vi "populate sonde row cluster from row.vi"(2 "Time Value":dbl, 7 "Initialize Initial Value Cluster":bool, 8 "error in (no error)":errorcluster, 9 "Sonde Parameters \nInitial Values":T3 {"Salinity Initial" format="%_2f"; "Temp Initial" format="%_2f"; "ORP  Initial" format="%_2f"; "pH Initial" format="%_2f"; "DO Initial" format="%_2f"; "SC Initial" format="%_2f"}, 10 "Array In":string[](array[string]), 11 "Sonde Parameters \nTolerance Limits":T6 {"Salinity %" format="%_2f%%"; "Temp %" format="%_2f%%"; "ORP %" format="%_2f%%"; "pH %" format="%_2f%%"; "DO %" format="%_2f%%"; "SC %" format="%_2f%%"}) -> (0 "error out":errorcluster, 1 "Cluster":T4 {"Salinity"."%" format="%_2f%%"; "Salinity"."Value" format="%_4g"; "Temperature"."%" format="%_2f%%"; "Temperature"."Value" format="%_4g"; "ORP"."%" format="%_2f%%"; "ORP"."Value" format="%_4g"; "pH"."%" format="%_2f%%"; "pH"."Value" format="%_4g"; "Dissolved Oxygen"."%" format="%_2f%%"; "Dissolved Oxygen"."Value" format="%_4g"; "Sp. Conductance"."%" format="%_2f%%"; "Sp. Conductance"."Value" format="%_4g"; "Cumulative\nVolume" format="%#_4g"}, 3 "Array out":string[](array[string]), 6 "Sonde Parameters \nInitial Values Out":T3 {"Salinity Initial" format="%_2f"; "Temp Initial" format="%_2f"; "ORP  Initial" format="%_2f"; "pH Initial" format="%_2f"; "DO Initial" format="%_2f"; "SC Initial" format="%_2f"})   [LabVIEW 2016]
uses:
  activeXtest/activeXtest 2015 Folder/sonde cluster from excel.ctl
  Sonde Value Percent Tol.ctl
  activeXtest/activeXtest 2015 Folder/sample data row cluster.ctl
  activeXtest/activeXtest 2015 Folder/sonde cluster.ctl
panel:
  in  "Sample Sheet Data Row Cluster":T1={"Head\nPressure"=0.0, "Depth"=0.0, "comment string"="", "Sonde Data Cluster"={"Cumulative\nVolume"=100.0, "Specific\nConductance"=2.0, "Dissolved\nOxygen"=3.0, "pH"=4.0, "ORP"=5.0, "Temp"=26.0, "Salinity"=7.0}} {"Sonde Data Cluster"."Salinity" format="%_3g"; "Sonde Data Cluster"."Temp" format="%_2g"; "Sonde Data Cluster"."ORP" format="%_4g"; "Sonde Data Cluster"."pH" format="%_4g"; "Sonde Data Cluster"."Dissolved\nOxygen" format="%_4g"; "Sonde Data Cluster"."Specific\nConductance" format="%_4g"; "Sonde Data Cluster"."Cumulative\nVolume" format="%#_4g"}
  in  "Input Cluster for % calculation":T4 caption="Cluster" {"Salinity"."%" format="%_2f%%"; "Salinity"."Value" format="%_4g"; "Temperature"."%" format="%_2f%%"; "Temperature"."Value" format="%_4g"; "ORP"."%" format="%_2f%%"; "ORP"."Value" format="%_4g"; "pH"."%" format="%_2f%%"; "pH"."Value" format="%_4g"; "Dissolved Oxygen"."%" format="%_2f%%"; "Dissolved Oxygen"."Value" format="%_4g"; "Sp. Conductance"."%" format="%_2f%%"; "Sp. Conductance"."Value" format="%_4g"; "Cumulative\nVolume" format="%#_4g"}
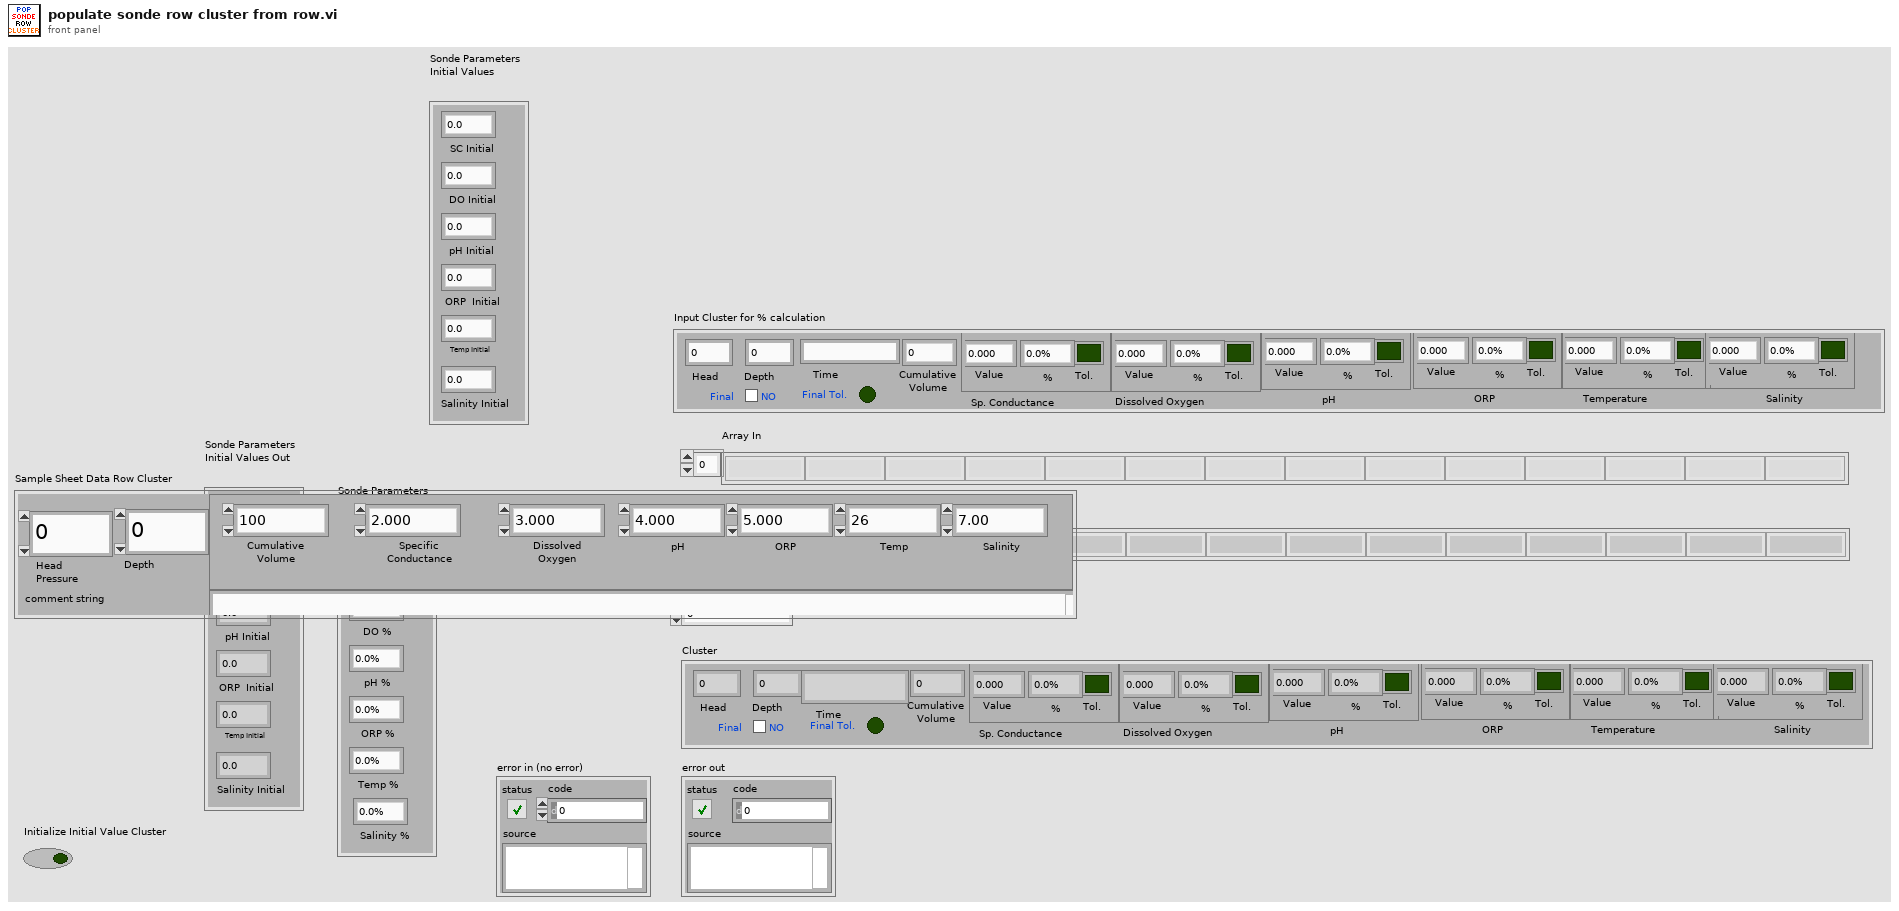
[diagram p1: front panel]
types:
  T1 = typedef "sample data row cluster.ctl" = cluster{"Head\nPressure":dbl, "Depth":dbl, "comment string":string, "Sonde Data Cluster":T2}
  T2 = typedef "sonde cluster.ctl" = cluster{"Cumulative\nVolume":dbl, "Specific\nConductance":dbl, "Dissolved\nOxygen":dbl, "pH":dbl, "ORP":dbl, "Temp":dbl, "Salinity":dbl}
  T3 = cluster{"SC Initial ":dbl, "DO Initial ":dbl, "pH Initial  ":dbl, "ORP  Initial":dbl, "Temp Initial":dbl, "Salinity Initial ":dbl}
  T4 = typedef "sonde cluster from excel.ctl" = cluster{"Head":dbl, "Depth":dbl, "Time":string, "Cumulative\nVolume":dbl, "Sp. Conductance":T5, "Dissolved Oxygen":T5, "pH":T5, "ORP":T5, "Temperature":T5, "Salinity":T5, "Final Tol.":bool, "Final":bool}
  T5 = typedef "Sonde Value Percent Tol.ctl" = cluster{"Value":dbl, "%":dbl, "Tol.":bool}
  T6 = cluster{"SC %":dbl, "DO %":dbl, "pH % ":dbl, "ORP % ":dbl, "Temp % ":dbl, "Salinity %":dbl}
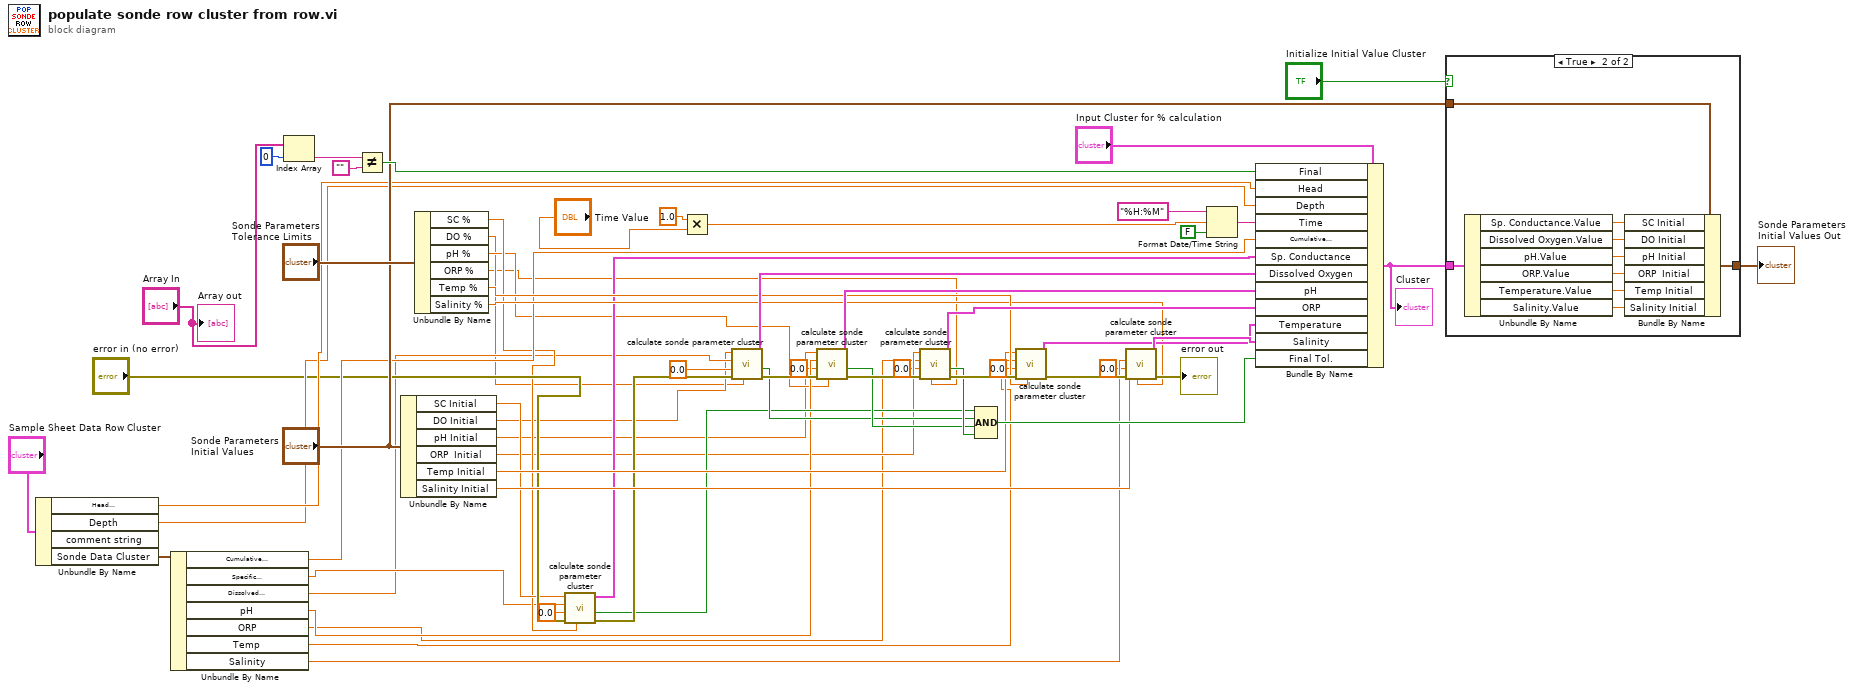
[diagram p0: block diagram]
diagram:
  n1 = Unbundle By Name("Sample Sheet Data Row Cluster") -> ("Head\nPressure"=w28:dbl, "Depth"=w27:dbl, "Sonde Data Cluster"=w26:T2)  [unwired: 1 out]
  n2 = Unbundle By Name(w26) -> ("Cumulative\nVolume"=w25:dbl, "Specific\nConductance"=w20:dbl, "Dissolved\nOxygen"=w14:dbl, "pH"=w16:dbl, "ORP"=w7:dbl, "Temp"=w4:dbl, "Salinity"=w2:dbl)
  n3 = Index Array(array="Array In", index=0) -> (element=w64:string)
  n4 = Not Equal?(x=w64, y="") -> (x != y?=w43:bool)
  n5 = Unbundle By Name("Sonde Parameters \nInitial Values") -> ("SC Initial"=w23:dbl, "DO Initial"=w12:dbl, "pH Initial"=w10:dbl, "ORP  Initial"=w8:dbl, "Temp Initial"=w34:dbl, "Salinity Initial"=w33:dbl)
  n6 = Unbundle By Name("Sonde Parameters \nTolerance Limits") -> ("SC %"=w22:dbl, "DO %"=w11:dbl, "pH %"=w15:dbl, "ORP %"=w6:dbl, "Temp %"=w40:dbl, "Salinity %"=w39:dbl)
  n7 = call "calculate sonde parameter cluster.vi"("tolerance limit"=w22, "error in (no error)"="error in (no error)", "Read % value"=0.0, "Read Value"=w20, "Initial Value"=w23) -> ("error out"=w19:errorcluster, "Tolerance"=w18:bool, "Cluster Out"=w21:T5)  [unwired: 3 in, 1 out]
  n8 = Multiply(x=1.0, y="Time Value") -> (x*y=w38:dbl)
  n9 = call "calculate sonde parameter cluster.vi"("tolerance limit"=w11, "error in (no error)"=w19, "Read % value"=0.0, "Read Value"=w14, "Initial Value"=w12) -> ("error out"=w61:errorcluster, "Tolerance"=w52:bool, "Cluster Out"=w47:T5)  [unwired: 3 in, 1 out]
  n10 = call "calculate sonde parameter cluster.vi"("tolerance limit"=w15, "error in (no error)"=w61, "Read % value"=0.0, "Read Value"=w16, "Initial Value"=w10) -> ("error out"=w60:errorcluster, "Tolerance"=w53:bool, "Cluster Out"=w48:T5)  [unwired: 3 in, 1 out]
  n11 = call "calculate sonde parameter cluster.vi"("tolerance limit"=w6, "error in (no error)"=w60, "Read % value"=0.0, "Read Value"=w7, "Initial Value"=w8) -> ("error out"=w59:errorcluster, "Tolerance"=w54:bool, "Cluster Out"=w49:T5)  [unwired: 3 in, 1 out]
  n12 = Compound Arithmetic op=AND(w18, w52, w53, w54) -> (w55:bool)
  n13 = call "calculate sonde parameter cluster.vi"("tolerance limit"=w40, "error in (no error)"=w59, "Read % value"=0.0, "Read Value"=w4, "Initial Value"=w34) -> ("error out"=w58:errorcluster, "Cluster Out"=w50:T5)  [unwired: 3 in, 2 out]
  n14 = call "calculate sonde parameter cluster.vi"("tolerance limit"=w39, "error in (no error)"=w58, "Read % value"=0.0, "Read Value"=w2, "Initial Value"=w33) -> ("error out"=→"error out":errorcluster, "Cluster Out"=w51:T5)  [unwired: 3 in, 2 out]
  n15 = Format Date/Time String(time format string (%c)="%H:%M", seconds (now)=w38, UTC format=FALSE) -> (date/time string=w46:string)
  n16 = Bundle By Name(cluster="Input Cluster for % calculation", "Final"=w43, "Head"=w28, "Depth"=w27, "Time"=w46, "Cumulative\nVolume"=w25, "Sp. Conductance"=w21, "Dissolved Oxygen"=w47, "pH"=w48, "ORP"=w49, "Temperature"=w50, "Salinity"=w51, "Final Tol."=w55) -> (w30:T4)
  "Cluster" <- w30
  n17 = case shown="True" "Initialize Initial Value Cluster" {
    tunnel: "Sonde Parameters \nInitial Values" -> [w65 w74]
    tunnel: [w65 w73] -> w32
    tunnel: w30 -> [_ w72]
    frame False {
    }
    frame True {
      n18 = Unbundle By Name(w72) -> ("Sp. Conductance.Value"=w71:dbl, "Dissolved Oxygen.Value"=w70:dbl, "pH.Value"=w69:dbl, "ORP.Value"=w68:dbl, "Temperature.Value"=w67:dbl, "Salinity.Value"=w66:dbl)
      n19 = Bundle By Name(cluster=w74, "SC Initial"=w71, "DO Initial"=w70, "pH Initial"=w69, "ORP  Initial"=w68, "Temp Initial"=w67, "Salinity Initial"=w66) -> (w73:T3)
    }
  }
  "Sonde Parameters \nInitial Values Out" <- w32
  "Array out" <- "Array In"
